vi "temp array gen start.vi"(7 "Temperature Control Parameters":T1 {"End Temp" format="%.2f"; "Temp Step" format="%.2f"; "Start Temp" format="%.2f"}) -> (4 "Temp Array":dbl[](array[numeric]), 10 "Warning time step too small":bool, 15 "N temps":i32)   [LabVIEW 2016]
doc: "This subvi checks if the parameters are in range, and if is too small sets a default value. Also, checks if the time step should be negative or positive depending of the input. The subvi returns an array with the correct parameters by performing some simple calculations in order to return the correct output.\n\nAlexis Lopez\nP350\nCSUSB Physics"
uses:
  typedefs/temp control params.ctl
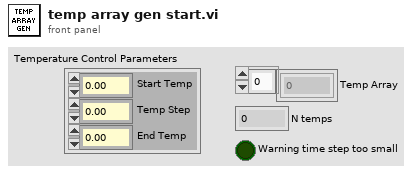
[diagram p1: front panel]
types:
  T1 = typedef "temp control params.ctl" = cluster{"Start Temp":dbl, "Temp Step":dbl, "End Temp":dbl}
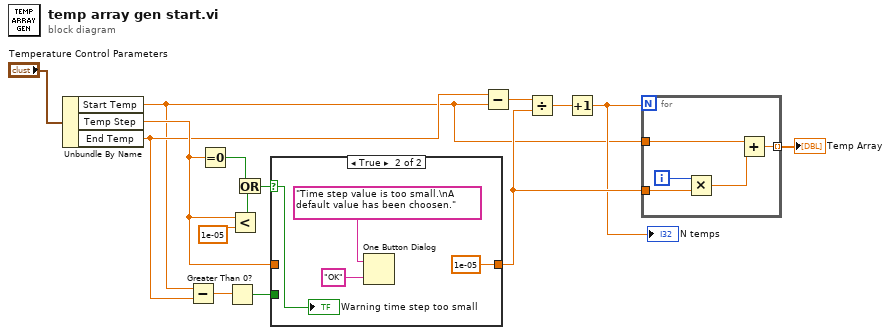
[diagram p0: block diagram]
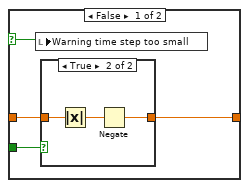
[diagram p2: hidden frame]
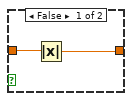
[diagram p3: hidden frame]
diagram:
  n1 = Unbundle By Name("Temperature Control Parameters") -> ("Start Temp"=w1:dbl, "Temp Step"=w4:dbl, "End Temp"=w2:dbl)
  n2 = Subtract(x=w1, y=w2) -> (x-y=w14:dbl)
  n3 = Equal To 0?(x=w4) -> (x = 0?=w5:bool)
  n4 = Greater Than 0?(x=w14) -> (x > 0?=w13:bool)
  n5 = Less?(x=w4, y=1e-05) -> (x < y?=w3:bool)
  n6 = Or(x=w5, y=w3) -> (x .or. y?=w6:bool)
  n7 = case shown="True" w6 {
    selector: w6 -> [w16 w25]
    tunnel: w4 -> [w18 _]
    tunnel: w13 -> [w19 _]
    tunnel: [w17 1e-05] -> w10
    frame False {
      n8 = local write "Warning time step too small"(w16) -> ()
      n9 = case shown="True" w19 {
        tunnel: w18 -> [w21 w24]
        tunnel: [w20 w22] -> w17
        frame False {
          n10 = Absolute Value(x=w21) -> (abs(x)=w20:dbl)
        }
        frame True {
          n11 = Absolute Value(x=w24) -> (abs(x)=w23:dbl)
          n12 = Negate(x=w23) -> (-x=w22:dbl)
        }
      }
    }
    frame True {
      n13 = One Button Dialog(message="Time step value is too small.\nA default value has been choosen.", button name ("OK")="OK") -> ()  [unwired: 1 out]
      "Warning time step too small" <- w25
    }
  }
  n14 = Subtract(x=w2, y=w1) -> (x-y=w12:dbl)
  n15 = Divide(x=w12, y=w10) -> (x/y=w11:dbl)
  n16 = Increment(x=w11) -> (x+1=w8:dbl)
  "N temps" <- w8
  n17 = for {
    N: w8 -> [_]
    tunnel: [w31] -> w9 mode=indexing
    tunnel: w10 -> [w30]
    tunnel: w1 -> [w29]
    i -> [w33]
    n18 = Multiply(x=w33, y=w30) -> (x*y=w32:dbl)
    n19 = Add(x=w29, y=w32) -> (x+y=w31:dbl)
  }
  "Temp Array" <- w9
